vi "KM101_MoveStoppedCallBack.vi"(4 "用户参数":variant, 5 "事件数据":cluster{"lChanID":i32}, 6 "控件引用":refnum<k7>, 7 "事件通用数据":cluster{"事件源":i32, "事件类型":u32, "时间标识":u32}) -> ()   [LabVIEW 2018, in "KIM101lib.lvlib"]
uses:
  KIM101lib.lvlib
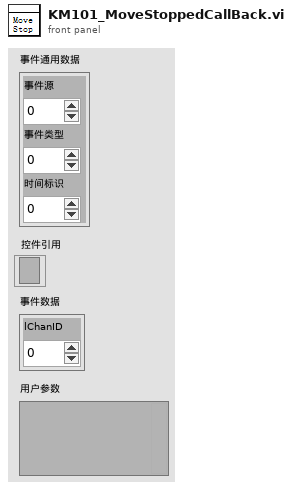
[diagram p1: front panel]
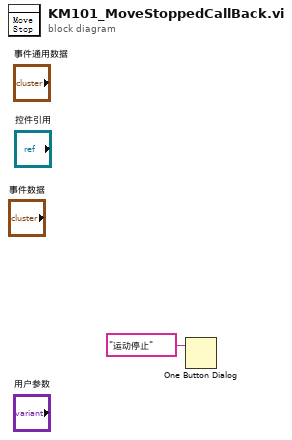
[diagram p0: block diagram]
diagram:
  n1 = One Button Dialog(message="运动停止" ("消息")) -> ()  [unwired: 1 in, 1 out]
